vi "Feed Controller.vi"(8 "error in":errorcluster) -> ()   [LabVIEW 2020]
doc: "This VI executes continuously carrying out the current operation and responding to updates or new operations. It will often contain the timing or control code that is difficult to place directly in TeleOp. This VI generally opens all sensors and motors and isolates the rest of the robot code from knowing how the operations are carried out."
uses:
  <vilib>/Rock Robotics/WPI/Framework/Completion Status.ctl
  Feed Setpoints.ctl
  Feed Operations.ctl
  <vilib>/Rock Robotics/SystemInterfaces/AI/FPGA_AIChannel.ctl
  <vilib>/Rock Robotics/WPI/ThirdParty/REV Robotics/REVLib/Typedef/Spark MAX Control Type.ctl
  <vilib>/Rock Robotics/Network Tables/NT Write Boolean.vi
panel:
  out "Voltage":dbl
  in  "BeamIsBroken?":bool
  in  "Interactive Values":T1
  out "Current\nCmd":string
  in  "Buttons":cluster{"Execute Cmd":bool, "Abort Cmd":bool}
  out "Command Timing":cluster{"Start Time (ms)":u32, "Iterations":i32}
  out "Status":T3
  # "Tip: It may be helpful to observe inputs and sensor values.\nYou may also want to display tuning or debugging controls."
  # "Interactive Command: You may fill in the settings for a command\nand schedule it with the Execute button. You can observe and abort\nany command while fine tuning the code for the controller."
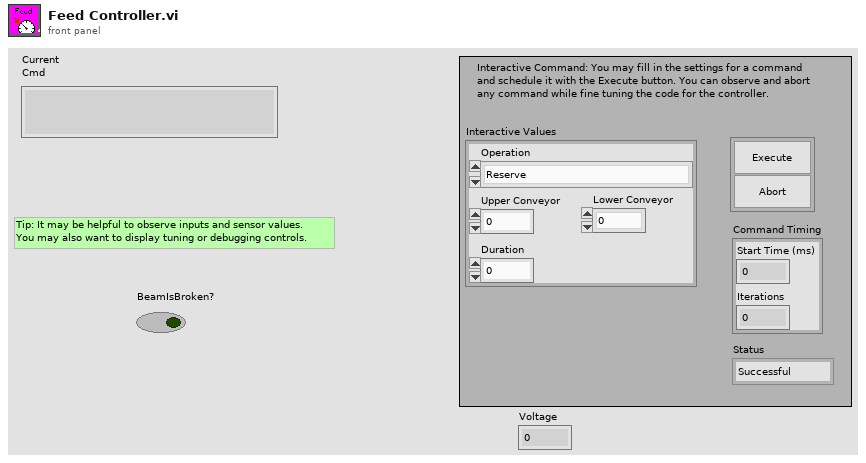
[diagram p1: front panel]
types:
  T1 = typedef "Feed Setpoints.ctl" = cluster{"Operation":T2, "Upper Conveyor":dbl, "Duration":dbl, "Lower Conveyor":dbl}
  T2 = typedef "Feed Operations.ctl" = enum16{"Reserve", "Read Current", "Immediate", "Feed For Time", "Feed For Sensor"}
  T3 = typedef "Completion Status.ctl" = enum16{"Successful", "Aborted", "Incomplete"}
  T4 = typedef "FPGA_AIChannel.ctl" = enum8{"AI 0", "AI 1", "AI 2", "AI 3", "AI MXP 0", "AI MXP 1", "AI MXP 2", "AI MXP 3", "Invalid"}
  T5 = typedef "WPI_AnalogChannelDevRef.ctl" = cluster{"DevStatus":errorcluster, "Analog Channel":T4}
  T6 = typedef "WPI_MotorControlDeviceRef.ctl" = cluster{"DeviceStatus":errorcluster, "Type":T7, "PWM":cluster{"PWM Channel":T8, "DeadBand":T9}, "CAN":cluster{"Device Number":u8, "SetOutput VI Ref":variant, "GetOutput VI Ref":variant, "Enable VI Ref":variant, "Disable VI Ref":variant, "Data":variant}, "Invert":bool, "DIO PWM":cluster{"PWM \"Enable\" Channel":T8, "DIOChannel":T10, "PWM Rate":dbl}}
  T7 = typedef "WPI_MotorControlType.ctl" = enum16{"PWM", "CAN", "DIO PWM"}
  T8 = typedef "FPGA_DIOPWMChannel.ctl" = enum8{"PWM 0", "PWM 1", "PWM 2", "PWM 3", "PWM 4", "PWM 5", "PWM 6", "PWM 7", "PWM 8", "PWM 9", "PWM MXP 0", "PWM MXP 1", "PWM MXP 2", "PWM MXP 3", "PWM MXP 4", "PWM MXP 5", "PWM MXP 6", "PWM MXP 7", "PWM MXP 8", "PWM MXP 9", "Invalid"}
  T9 = typedef "WPI_PWMDeadband.ctl" = cluster{"Name":string, "maxPositivePwm":i32, "minPositivePwm":i32, "centerPwm":i32, "maxNegativePwm":i32, "minNegativePwm":i32, "angularRange":u16}
  T10 = typedef "FPGA_DIOChannel.ctl" = enum8{"DIO 0", "DIO 1", "DIO 2", "DIO 3", "DIO 4", "DIO 5", "DIO 6", "DIO 7", "DIO 8", "DIO 9", "DIO MXP 0", "DIO MXP 1", "DIO MXP 2", "DIO MXP 3", "DIO MXP 4", "DIO MXP 5", "DIO MXP 6", "DIO MXP 7", "DIO MXP 8", "DIO MXP 9", "DIO MXP 10", "DIO MXP 11", "DIO MXP 12", "DIO MXP 13", "DIO MXP 14", "DIO MXP 15", "SPI Port CS1", "SPI Port CS2", "SPI Port CS3", "SPI Port MISO", "SPI Port MOSI", "Invalid"}
  T11 = typedef "Command Status Info.ctl" = cluster{"Name":string, "Status":T3, "notifier out":T12}
  T12 = typedef "Completion Notifier.ctl" = refnum<notifier>
  T13 = cluster{"Current Command":T1, "Command Timing":cluster{"Start Time (ms)":u32, "Iterations":i32}, "Command Arguments":cluster{"Command Info":T11, "Description":string, "Default Command":T1, "queue out":refnum<queue>, "Subsystem Name":string}}
  T14 = typedef "Spark MAX Control Type.ctl" = enum16{"Percent VBus", "Voltage", "Velocity", "Position", "Smart Motion", "Current", "Smart Velocity"}
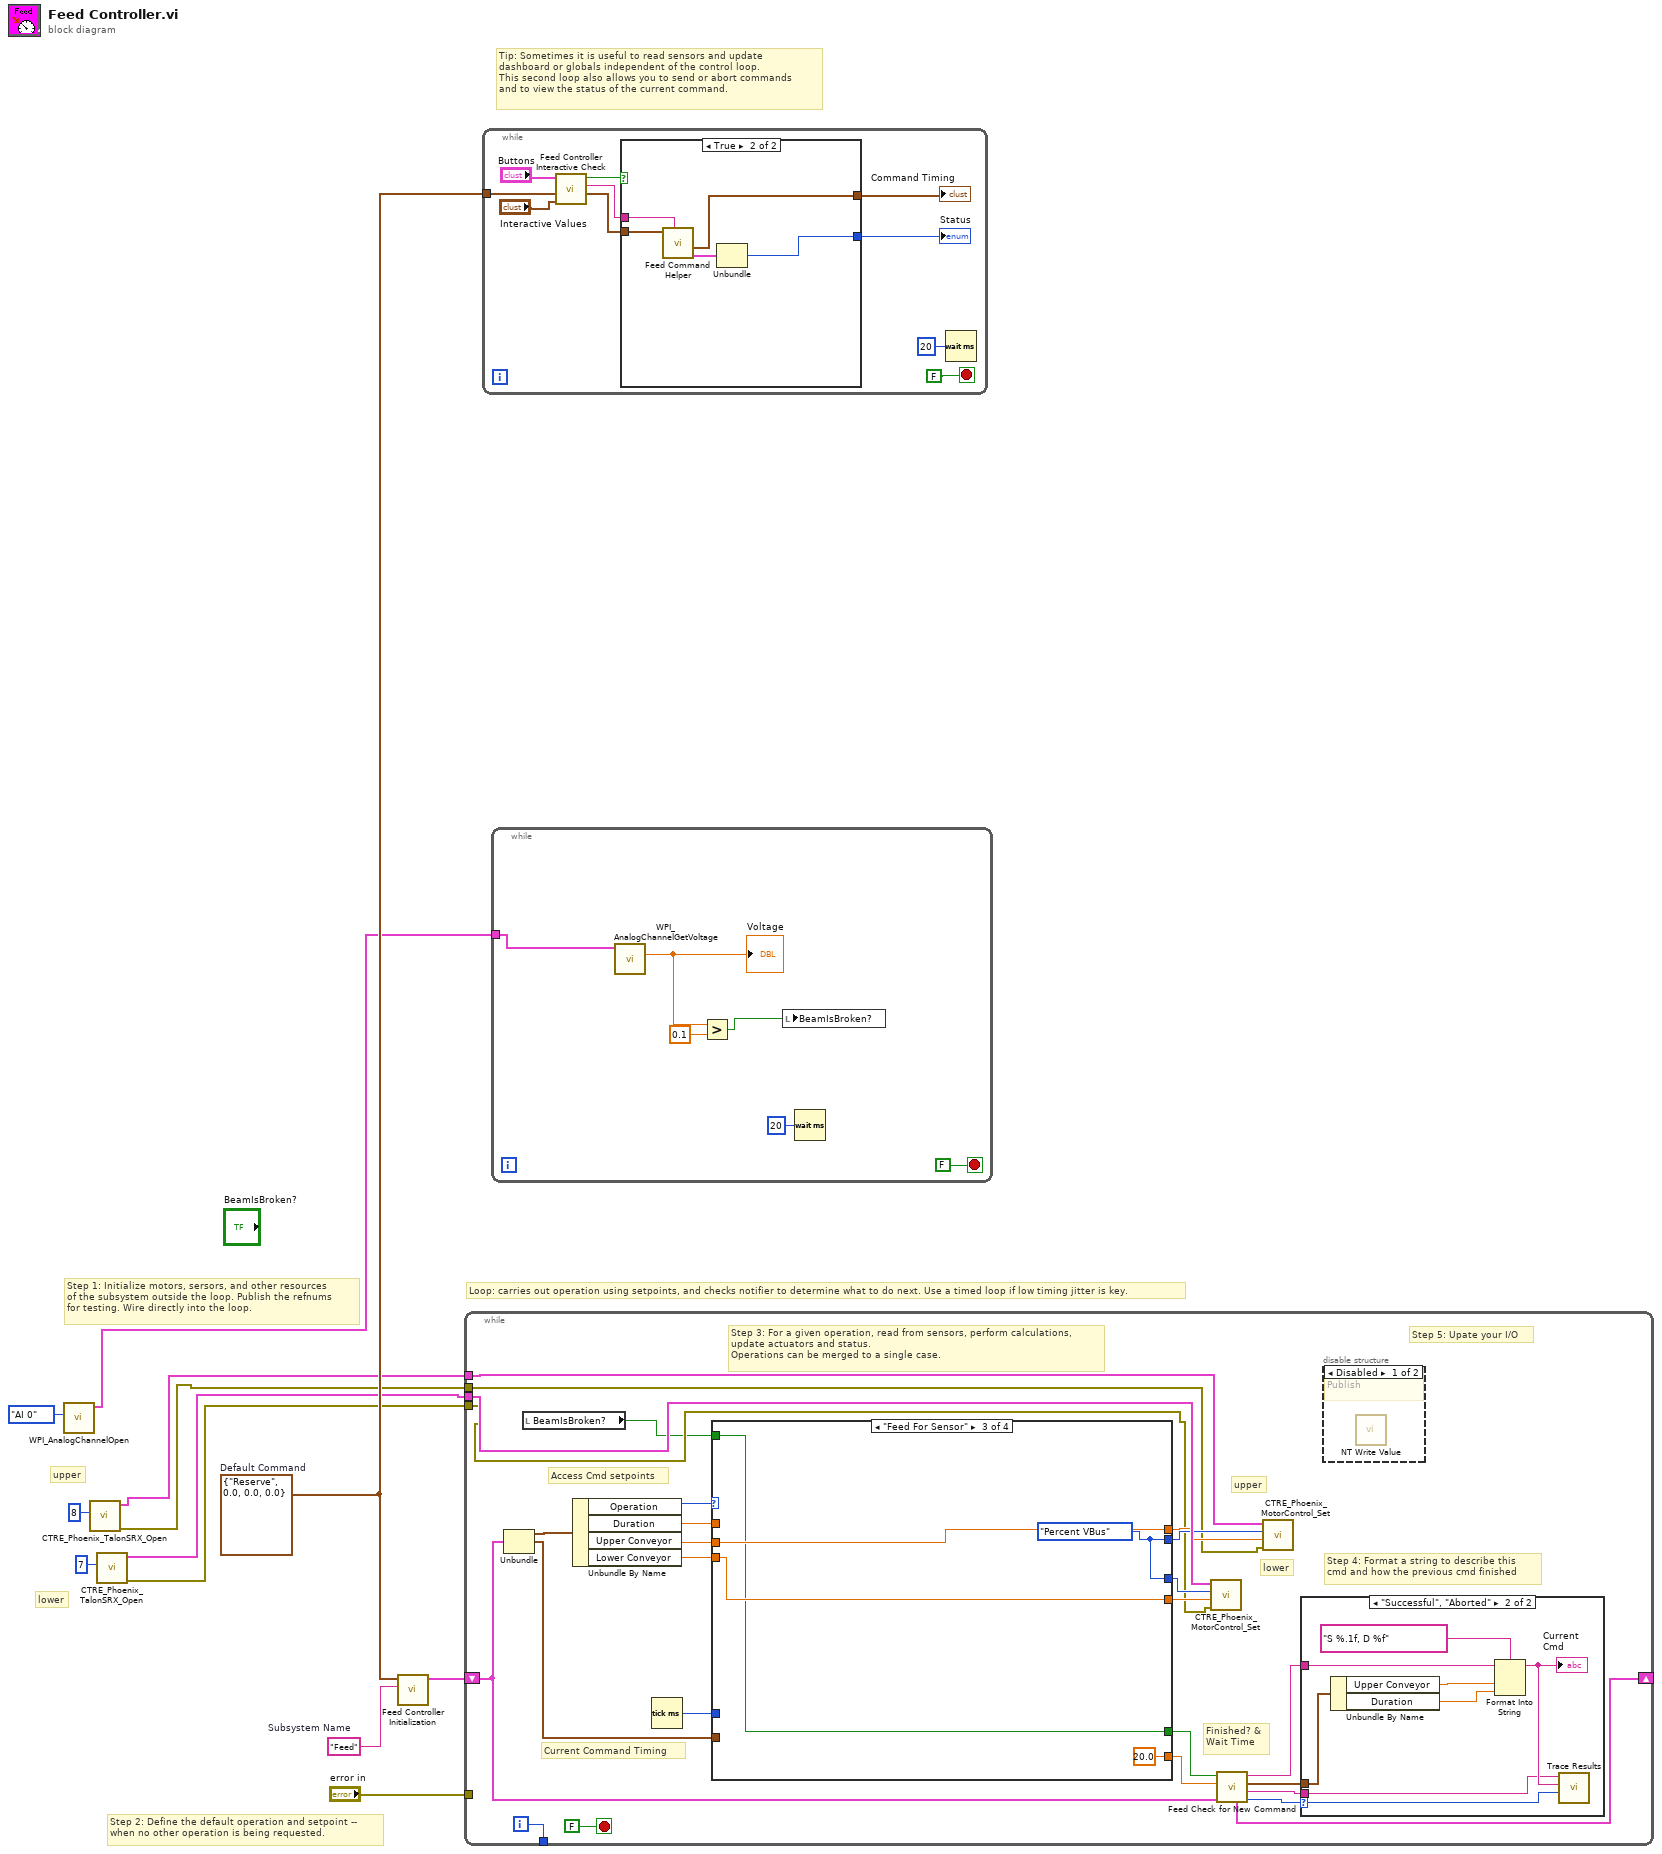
[diagram p0: block diagram]
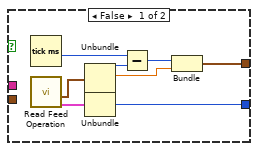
[diagram p2: hidden frame]
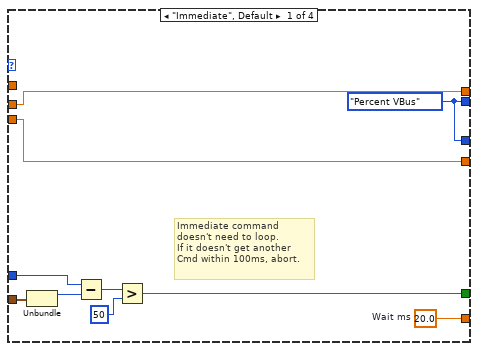
[diagram p5: hidden frame]
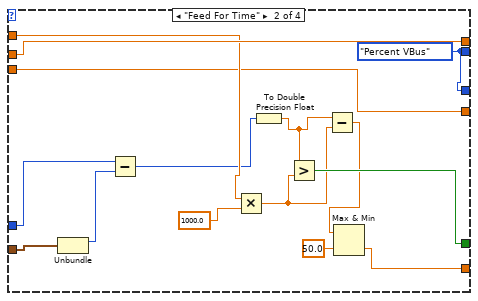
[diagram p6: hidden frame]
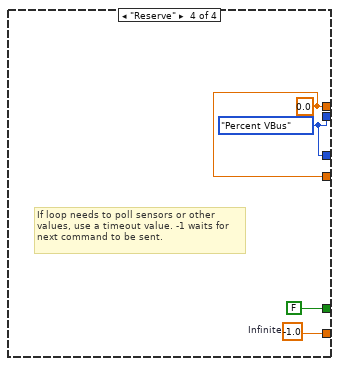
[diagram p7: hidden frame]
diagram:
  w9 = T1 {"Operation"=enum."Reserve", "Upper Conveyor"=0.0, "Duration"=0.0, "Lower Conveyor"=0.0}  # Default Command
  w10 = "Feed"  # Subsystem Name
  # "lower"
  # "upper"
  # "Tip: Sometimes it is useful to read sensors and update\ndashboard or globals independent of the control loop.\nThis second loop also allows you to send or abort commands\nand to view the status of the current command."
  # "Step 2: Define the default operation and setpoint --\nwhen no other operation is being requested."
  # "Step 1: Initialize motors, sersors, and other resources\nof the subsystem outside the loop. Publish the refnums\nfor testing. Wire directly into the loop."
  # "Loop: carries out operation using setpoints, and checks notifier to determine what to do next. Use a timed loop if low timing jitter is key."
  n1 = call <vilib>:"WPI_AnalogChannelOpen.vi"("Analog Channel"=FPGA_AIChannel."AI 0") -> ("AIDeviceRef"=w1:T5)  [unwired: 9 in, 1 out]
  n2 = call <vilib>:"CTRE_Phoenix_TalonSRX_Open.vi"("Device Number"=u8 8) -> ("error out"=w3:errorcluster, "PhoenixMotorControlDevRef"=w8:T6)  [unwired: 9 in]
  n3 = call <vilib>:"CTRE_Phoenix_TalonSRX_Open.vi"("Device Number"=u8 7) -> ("error out"=w4:errorcluster, "PhoenixMotorControlDevRef"=w5:T6)  [unwired: 9 in]
  n4 = call "Feed Controller Initialization.vi"("Subsystem Name"=w10, "Default Command"=w9) -> ("Current Command"=w11:T13)  [unwired: 9 in]
  n5 = while {
    shift-right: [w30] -> _
    shift-left: w11 -> [w23]
    tunnel: [w37] -> _
    tunnel: "error in" -> [_]
    tunnel: w8 -> [w21]
    tunnel: w5 -> [w20]
    tunnel: w4 -> [w15]
    tunnel: w3 -> [w14]
    i -> [w37]
    stop <- FALSE stop-if-true
    # "lower"
    # "upper"
    # "Step 5: Upate your I/O"
    # "Step 4: Format a string to describe this\ncmd and how the previous cmd finished"
    # "Current Command Timing"
    # "Access Cmd setpoints"
    # "Finished? &\nWait Time"
    # "Step 3: For a given operation, read from sensors, perform calculations,\nupdate actuators and status.\nOperations can be merged to a single case."
    n6 = Unbundle(w23) -> ("Current Command"=w36:T1, "Command Timing"=w32:cluster{"Start Time (ms)":u32, "Iterations":i32})  [unwired: 1 out]
    n7 = local read "BeamIsBroken?"() -> (w13:bool)
    n8 = Unbundle By Name(w36) -> ("Operation"=w35:T2, "Duration"=w34:dbl, "Upper Conveyor"=w31:dbl, "Lower Conveyor"=w22:dbl)
    n9 = Tick Count (ms)() -> (millisecond timer value=w33:u32)
    n10 = case shown="\"Feed For Sensor\"" w35 {
      tunnel: [w56 w59 20.0 ("Infinite") w80] -> w28
      tunnel: [w51 w68 w72 FALSE ("ignore previous (F)")] -> w29
      tunnel: w32 -> [w53 w70 _ _]
      tunnel: w34 -> [_ w66 _ _]
      tunnel: w33 -> [w52 w69 _ _]
      tunnel: w31 -> [w50 w71 w76 _]
      tunnel: [w50 w71 w76 w77] -> w17
      tunnel: [w47 w57 w73 w78] -> w18
      tunnel: w22 -> [w48 w58 w74 _]
      tunnel: [w48 w58 w74 w77] -> w19
      tunnel: [w47 w57 w73 w78] -> w16
      tunnel: w13 -> [_ _ w72 _]
      frame "Immediate", Default {
        w47 = Spark_MAX_Control_Type."Percent VBus" ("Control Mode")
        w56 = 20.0  # Wait ms
        # "Immediate command\ndoesn't need to loop.\nIf it doesn't get another\nCmd within 100ms, abort."
        n11 = Unbundle(w53) -> ("Start Time (ms)"=w55:u32)  [unwired: 1 out]
        n12 = Subtract(x=w52, y=w55) -> (x-y=w54:u32)
        n13 = Greater?(x=w54, y=u32 50) -> (0:w51:bool)
      }
      frame "Feed For Time" {
        w57 = Spark_MAX_Control_Type."Percent VBus" ("Control Mode")
        n14 = Unbundle(w70) -> ("Start Time (ms)"=w67:u32)  [unwired: 1 out]
        n15 = Subtract(x=w69, y=w67) -> (x-y=w64:u32)
        n16 = Multiply(x=w66, y=1000.0) -> (x*y=w62:dbl)
        n17 = To Double Precision Float(number=w64) -> (double precision float=w61:dbl)
        n18 = Greater?(x=w61, y=w62) -> (0:w68:bool)
        n19 = Subtract(x=w61, y=w62) -> (x-y=w60:dbl)
        n20 = Max & Min(x=w60, y=50.0) -> (min(x,y)=w59:dbl)  [unwired: 1 out]
      }
      frame "Feed For Sensor" {
        w73 = Spark_MAX_Control_Type."Percent VBus" ("Control Mode")
      }
      frame "Reserve" {
        w78 = Spark_MAX_Control_Type."Percent VBus" ("Control Mode")
        w77 = 0.0 ("Setpoint")
        w80 = -1.0  # Infinite
        # "If loop needs to poll sensors or other\nvalues, use a timeout value. -1 waits for\nnext command to be sent."
      }
    }
    n21 = call <vilib>:"CTRE_Phoenix_MotorControl_Set.vi"("error in (no error)"=w15, "Output"=w19, "Control Mode"=w16, "PhoenixMotorControlDevRef"=w20) -> ()  [unwired: 6 in, 2 out]
    n22 = call "Feed Check for New Command.vi"("Current Command"=w23, "Wait time (ms)"=w28, "Finished?"=w29) -> ("Completion"=w24:T3, "Subsystem Name"=w25:string, "Current Command"=w26:T1, "Initial Trace String"=w27:string, "NextCommand"=w30:T13)  [unwired: 4 in]
    n23 = call <vilib>:"CTRE_Phoenix_MotorControl_Set.vi"("error in (no error)"=w14, "Output"=w17, "Control Mode"=w18, "PhoenixMotorControlDevRef"=w21) -> ()  [unwired: 6 in, 2 out]
    n24 = case shown="\"Successful\", \"Aborted\"" w24 {
      selector: w24 -> [_ w46]
      tunnel: w27 -> [_ w42]
      tunnel: w26 -> [_ w43]
      tunnel: w25 -> [_ w39]
      frame "Incomplete", Default {
        # "Continuing current command"
      }
      frame "Successful", "Aborted" {
        # "Report and setup for next command"
        n25 = Unbundle By Name(w43) -> ("Upper Conveyor"=w45:dbl, "Duration"=w40:dbl)
        n26 = Format Into String(format string="S %.1f, D %f", initial string=w42, w45, w40) -> (resulting string=w41:string)  [unwired: 1 in, 1 out]
        "Current\nCmd" <- w41
        n27 = call <vilib>:"Trace Results.vi"("Status of previous command"=w46, "Description"=w41, "Subsystem"=w39) -> ()  [unwired: 9 in]
      }
    }
    n28 = disable-structure shown="Disabled" {
      frame Disabled {
        # "Publish"
        n29 = call-poly <vilib>:"NT Write Value.vi"() -> ()  [unwired: 11 in, 1 out]
      }
      frame Enabled {
      }
    }
  }
  n30 = while {
    tunnel: w9 -> [w87]
    stop <- FALSE stop-if-true
    n31 = call "Feed Controller Interactive Check.vi"("Interactive Command in"="Interactive Values", "Default Command"=w87, "Buttons"="Buttons") -> ("Interactive Command out"=w84:T1, "Trace String"=w85:string, "Schedule"=w86:bool)  [unwired: 6 in]
    n32 = case shown="True" w86 {
      tunnel: [w98 w103] -> w83
      tunnel: w84 -> [_ w101]
      tunnel: [w94 w99] -> w82
      tunnel: w85 -> [_ w102]
      frame False {
        n33 = Tick Count (ms)() -> (millisecond timer value=w93:u32)
        n34 = call "Read Feed Operation.vi"() -> ("Command Info"=w91:T11, "SubSystem Data"=w92:T1)  [unwired: 9 in, 1 out]
        n35 = Unbundle(w92) -> ("Operation"=w97:T2, "Upper Conveyor"=w95:dbl)  [unwired: 2 out]
        n36 = Unbundle(w91) -> ("Status"=w98:T3)  [unwired: 2 out]
        n37 = Subtract(x=w93, y=w97) -> (x-y=w96:u32)
        n38 = Bundle(w96, "Upper Conveyor"=w95) -> (w94:cluster{u32, "Upper Conveyor":dbl})  [unwired: 1 in]
      }
      frame True {
        n39 = call "Feed Command Helper.vi"("Description"=w102, "SubSystem Data"=w101) -> ("Command Info Out"=w100:T11, "Command Timing"=w99:cluster{"Start Time (ms)":u32, "Iterations":i32})  [unwired: 7 in, 1 out]
        n40 = Unbundle(w100) -> ("Status"=w103:T3)  [unwired: 2 out]
      }
    }
    "Status" <- w83
    "Command Timing" <- w82
    n41 = Wait (ms)(milliseconds to wait=u32 20) -> ()  [unwired: 1 out]
  }
  n42 = while {
    tunnel: w1 -> [w107]
    stop <- FALSE stop-if-true
    n43 = call <vilib>:"WPI_AnalogChannelGetVoltage.vi"("AIDeviceRef"=w107) -> ("Voltage"=w106:dbl)  [unwired: 8 in, 2 out]
    "Voltage" <- w106
    n44 = Greater?(x=w106, y=0.1) -> (0:w104:bool)
    n45 = local write "BeamIsBroken?"(w104) -> ()
    n46 = Wait (ms)(milliseconds to wait=u32 20) -> ()  [unwired: 1 out]
  }
